vi "toml_parse_element.vi"(8 "error in (no error)":errorcluster, 11 "string":string) -> (0 "error out":errorcluster, 2 "value":variant, 3 "remaining string":string)   [LabVIEW 2017]
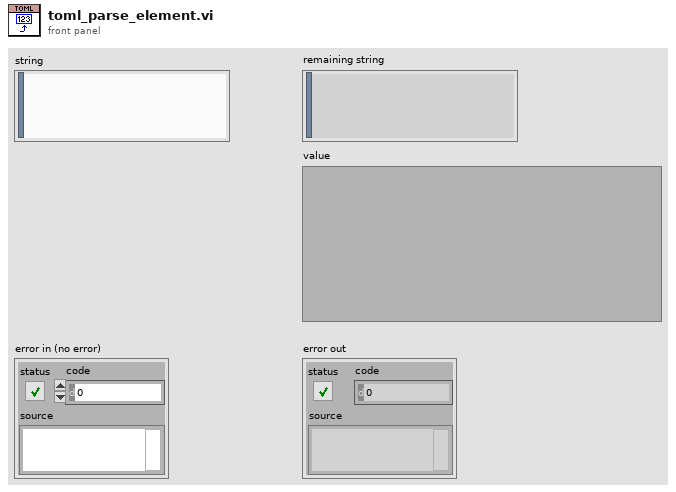
[diagram p1: front panel]
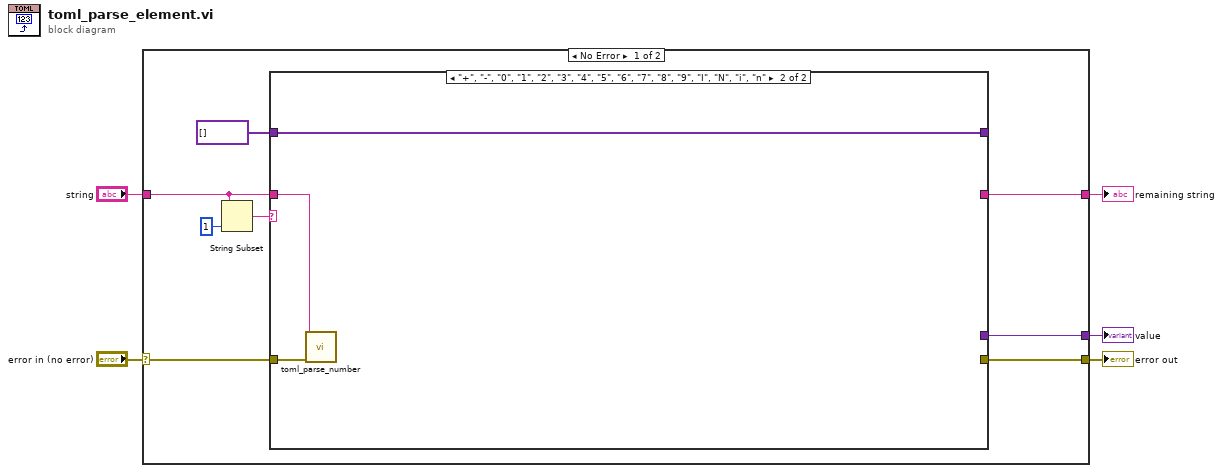
[diagram p0: block diagram]
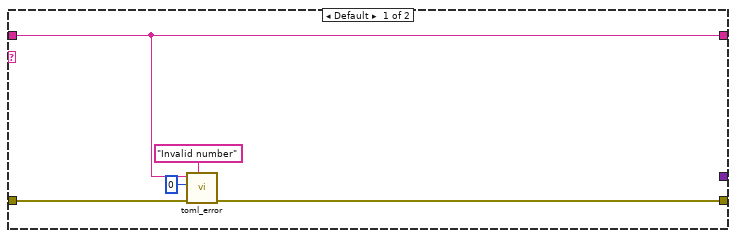
[diagram p2: hidden frame]
diagram:
  n1 = case shown="No Error" "error in (no error)" {
    selector: "error in (no error)" -> [w13 w23]
    tunnel: "string" -> [w12 w22]
    tunnel: [w10 w23] -> w3
    tunnel: [w8 w22] -> w2
    tunnel: [w7 _] -> w1
    frame No Error {
      n2 = String Subset(string=w12, length (rest)=1 ("length (rest)")) -> (substring=w9:string)  [unwired: 1 in]
      n3 = case shown="\"+\", \"-\", \"0\", \"1\", \"2\", \"3\", \"4\", \"5\", \"6\", \"7\", \"8\", \"9\", \"I\", \"N\", \"i\", \"n\"" w9 {
        tunnel: w13 -> [w18 w21]
        tunnel: w12 -> [w16 w19]
        tunnel: [w17 _] -> w10
        tunnel: [w16 _] -> w8
        tunnel: [_ _] -> w7
        tunnel: [_ w20] -> _
        tunnel: variant[] [] -> [_ w20]
        frame Default {
          n4 = call "toml_error.vi"("message"="Invalid number" ("source"), "error in (no error)"=w18, "offset (0)"=0, "toml"=w16) -> ("error out"=w17:errorcluster)  [unwired: 7 in]
        }
        frame "+", "-", "0", "1", "2", "3", "4", "5", "6", "7", "8", "9", "I", "N", "i", "n" {
          n5 = call "toml_parse_number.vi"("error in (no error)"=w21, "string"=w19) -> ()  [unwired: 7 in, 3 out]
        }
      }
    }
    frame Error {
    }
  }
  "error out" <- w3
  "remaining string" <- w2
  "value" <- w1
